vi "Escape parens and backslashes.vi"(7 "Input String":string) -> (8 "Escaped String":string)   [LabVIEW 2018, in "Path and String Processing.lvlib"]
uses:
  Path and String Processing.lvlib
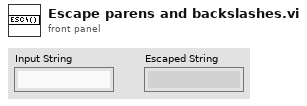
[diagram p1: front panel]
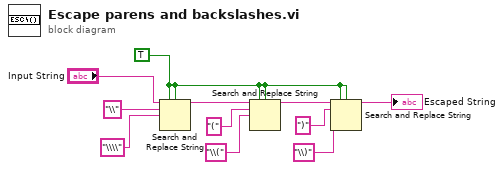
[diagram p0: block diagram]
diagram:
  w11 = TRUE ("replace all? (F)")
  n1 = Search and Replace String(replace all?=w11, case sensitive?=w11, input string="Input String", search string="\\", replace string="\\\\" ("replace string (\"\")")) -> (result string=w6:string)  [unwired: 3 in, 3 out]
  n2 = Search and Replace String(replace all?=w11, case sensitive?=w11, input string=w6, search string="(", replace string="\\(" ("replace string (\"\")")) -> (result string=w9:string)  [unwired: 3 in, 3 out]
  n3 = Search and Replace String(replace all?=w11, case sensitive?=w11, input string=w9, search string=")", replace string="\\)" ("replace string (\"\")")) -> (result string=→"Escaped String":string)  [unwired: 3 in, 3 out]
